vi "Print CD Error.vi"(5 "Custom Device? (T)":bool=TRUE, 7 "error out":errorcluster, 10 "Your code's public name":string) -> ()   [LabVIEW 2010, in "Agilent 364xA (GPIB,Serial) Custom Device.lvlib"]
doc: "Prints error information out to the console. Provide your code's public name. For example, if your code is about J1939, put that here so the user knows what this printed error information has to do with.\n\nIf this is not a NI VeriStand custom device, write false to the Custom Device? input. This will change the error output.\n\nIf the 'note' field is empty, it is not printed to the console.\n\nExample output 1:\n******J1939 ERROR******\nSource: blah.vi\nCode: 535\n******J1939 ERROR******\n\nExample output 2:\n******XCP and CCP Master CUSTOM DEVICE ERROR******\nSource: blah.vi\nCode: 535\nUser Note: before write\n******XCP and CCP Master CUSTOM DEVICE ERROR******"
uses:
  <vilib>/Utility/error.llb/DialogType.ctl
  Agilent 364xA (GPIB,Serial) Custom Device.lvlib
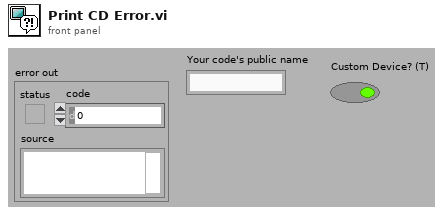
[diagram p1: front panel]
types:
  T1 = typedef "DialogType.ctl" = u16
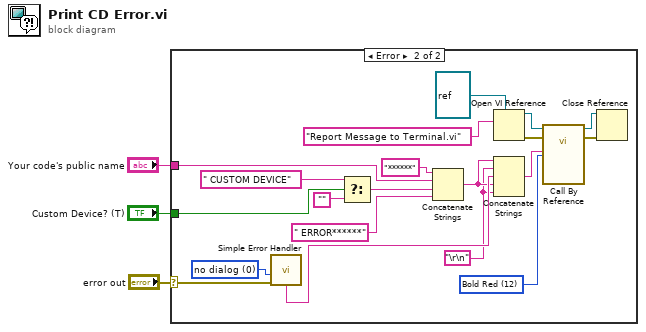
[diagram p0: block diagram]
diagram:
  n1 = case shown="Error" "error out" {
    selector: "error out" -> [_ w9]
    tunnel: "Custom Device? (T)" -> [_ w18]
    tunnel: "Your code's public name" -> [_ w4]
    frame No Error {
    }
    frame Error {
      w8 = T1 0 items=["no dialog", "OK message", "continue or stop message", "OK message + warnings", "continue/stop + warnings"] ("type of dialog (OK msg:1)")
      w10 = u16 12 items=["Plain White"=7, "Bold White"=15, "Bold Blue"=9, "Bold Green"=10, "Bold Red"=12] ("Color (Plain White)")
      w5 = "\r\n"
      n2 = call <vilib>:"Simple Error Handler.vi"("type of dialog (OK msg:1)"=w8, "error in (no error)"=w9) -> ("message"=w7:string)  [unwired: 3 in, 4 out]
      n3 = Select(t=" CUSTOM DEVICE" ("String"), s=w18, f="") -> (s? t:f=w19:string)
      n4 = Concatenate Strings("******" ("String"), w4, w19, " ERROR******" ("String")) -> (w6:string)
      n5 = Open VI Reference(type specifier VI Refnum (for type only)=refnum<vi> refnum, vi path="Report Message to Terminal.vi") -> (vi reference=w15:refnum<vi>, error out=w14:errorcluster)  [unwired: 1 in, 3 out]
      n6 = Concatenate Strings(w6, w5, w7, w6, w5) -> (w11:string)
      n7 = call-by-ref "?"(reference=w15, error in=w14, "Color (Plain White)"=w10, "Message"=w11) -> (reference out=w12:refnum<vi>, error out=w13:errorcluster)  [unwired: 9 in, 1 out]
      n8 = Close Reference(reference=w12, error in (no error)=w13) -> ()  [unwired: 1 out]
    }
  }
